vi "trimspace non-reentrant vs reentrant vs inline.vi"() -> ()   [LabVIEW 2020]
panel:
  out "inside 3":i32
  out "[\\t\\n\\r\\s] 2":string
  out "outside 3":i32
  out "[\\t\\n\\r\\s]":string
  out "[\\t\\s]":string
  out "inside 2":i32
  out "outside 2":i32
  out "inside":i32
  out "outside":i32
  out "unit (ms)":dbl[][](graph)
  # "non-reentrant"
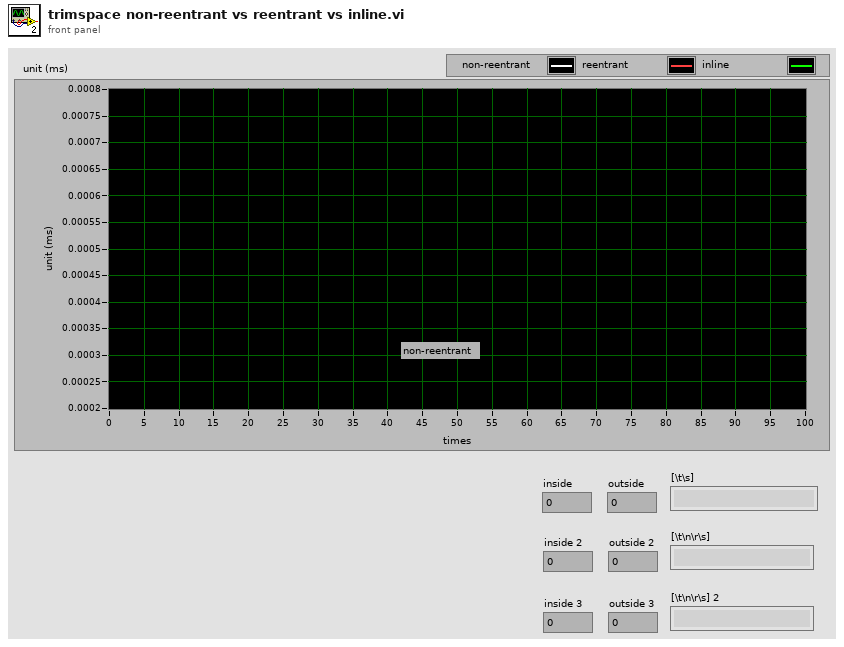
[diagram p1: front panel]
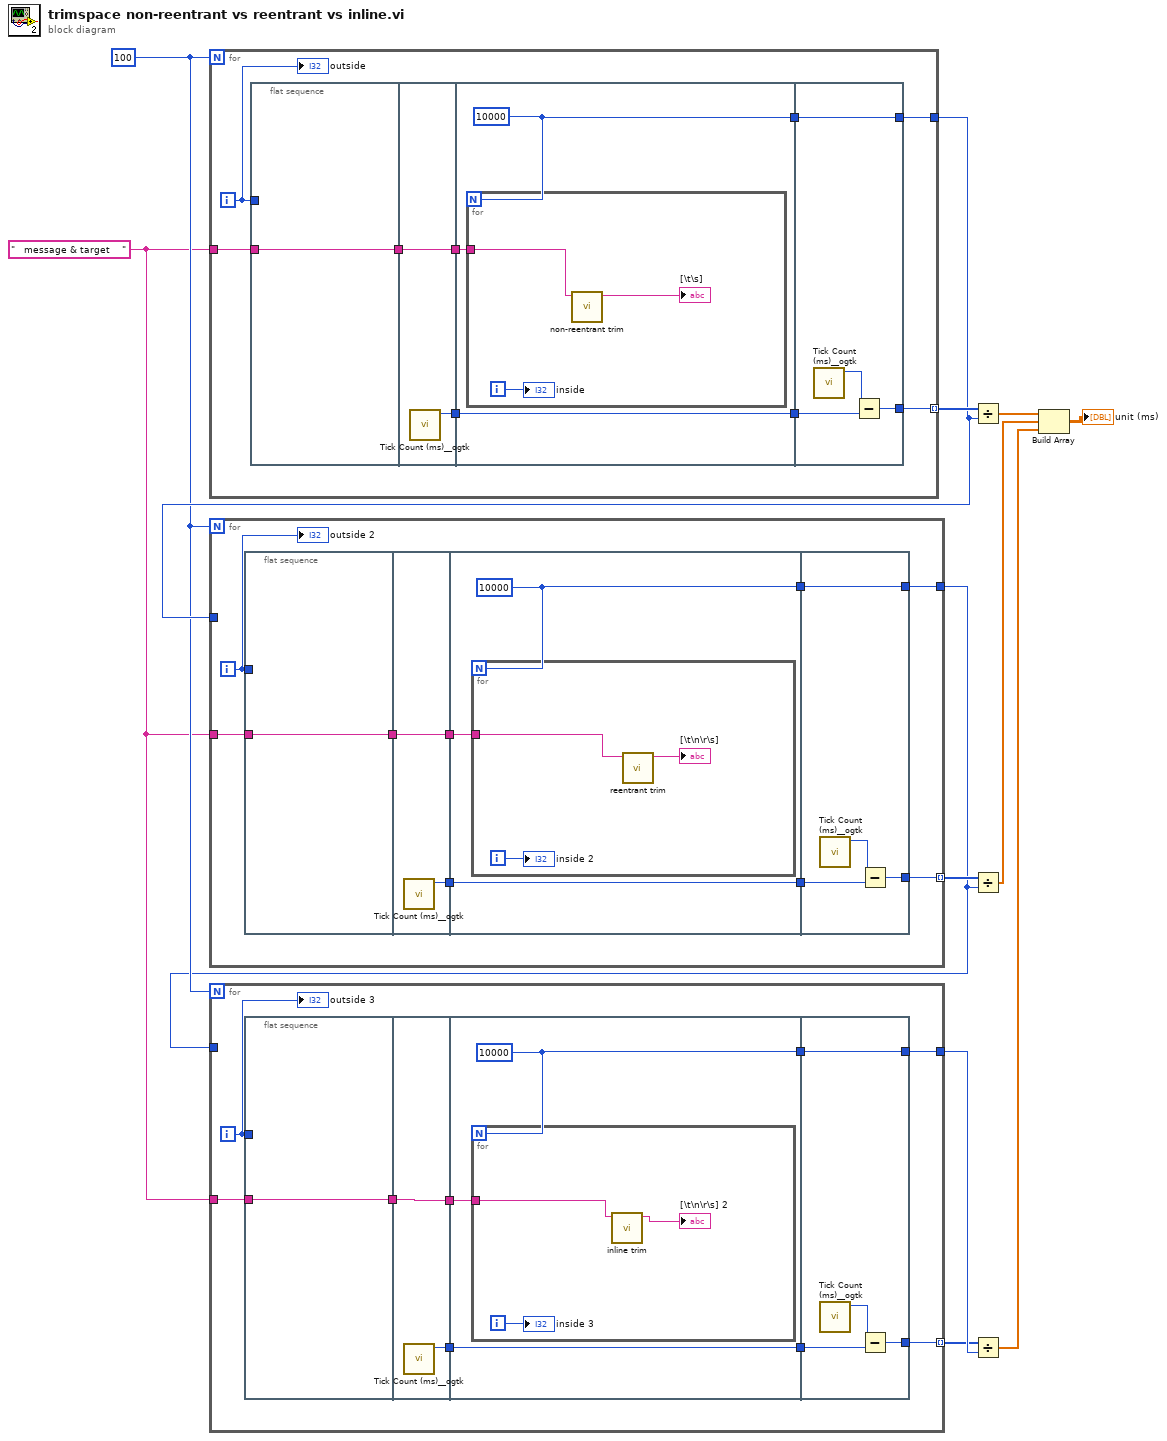
[diagram p0: block diagram]
diagram:
  w2 = "   message & target    " ("string")
  w4 = 100
  n1 = for {
    N: w4 -> [_]
    tunnel: [w19] -> w12 mode=indexing
    tunnel: [w18] -> w9
    tunnel: w2 -> [w13]
    i -> [w16]
    n2 = flat-sequence {
      tunnel: w16 -> [_]
      tunnel: [w22] -> w14
      tunnel: w13 -> [w22]
      tunnel: [w24] -> w21
      tunnel: [w23] -> w15
      tunnel: w14 -> [w23]
      tunnel: w21 -> [w27]
      tunnel: [w27] -> w20
      tunnel: [w26] -> w17
      tunnel: w15 -> [w25]
      tunnel: w20 -> [w33]
      tunnel: [w32] -> w19
      tunnel: [w31] -> w18
      tunnel: w17 -> [w31]
      frame #0 {
      }
      frame #1 {
        n3 = call <userlib>:"Tick Count (ms)__ogtk.vi"() -> ("millisecond timer value"=w24:u32)  [unwired: 10 in, 1 out]
      }
      frame #2 {
        w26 = 10000
        n4 = for {
          N: w26 -> [_]
          tunnel: w25 -> [w29]
          i -> [w30]
          n5 = call "non-reentrant trim.vi"("string in"=w29) -> ("string out"=→"[\\t\\s]":string)  [unwired: 10 in]
          "inside" <- w30
        }
      }
      frame #3 {
        n6 = call <userlib>:"Tick Count (ms)__ogtk.vi"() -> ("millisecond timer value"=w34:u32)  [unwired: 10 in, 1 out]
        n7 = Subtract(x=w34, y=w33) -> (x-y=w32:u32)
      }
    }
    "outside" <- w16
  }
  n8 = for {
    N: w4 -> [_]
    tunnel: [w41] -> w10 mode=indexing
    tunnel: [w40] -> w3
    tunnel: w9 -> [_]
    tunnel: w2 -> [w35]
    i -> [w38]
    n9 = flat-sequence {
      tunnel: w38 -> [_]
      tunnel: [w44] -> w36
      tunnel: w35 -> [w44]
      tunnel: [w46] -> w43
      tunnel: [w45] -> w37
      tunnel: w36 -> [w45]
      tunnel: w43 -> [w49]
      tunnel: [w49] -> w42
      tunnel: [w48] -> w39
      tunnel: w37 -> [w47]
      tunnel: w42 -> [w55]
      tunnel: [w54] -> w41
      tunnel: [w53] -> w40
      tunnel: w39 -> [w53]
      frame #0 {
      }
      frame #1 {
        n10 = call <userlib>:"Tick Count (ms)__ogtk.vi"() -> ("millisecond timer value"=w46:u32)  [unwired: 10 in, 1 out]
      }
      frame #2 {
        w48 = 10000
        n11 = for {
          N: w48 -> [_]
          tunnel: w47 -> [w50]
          i -> [w52]
          n12 = call "reentrant trim.vi"("string in"=w50) -> ("string out"=→"[\\t\\n\\r\\s]":string)  [unwired: 10 in]
          "inside 2" <- w52
        }
      }
      frame #3 {
        n13 = call <userlib>:"Tick Count (ms)__ogtk.vi"() -> ("millisecond timer value"=w56:u32)  [unwired: 10 in, 1 out]
        n14 = Subtract(x=w56, y=w55) -> (x-y=w54:u32)
      }
    }
    "outside 2" <- w38
  }
  n15 = for {
    N: w4 -> [_]
    tunnel: [w63] -> w5 mode=indexing
    tunnel: [w62] -> w6
    tunnel: w2 -> [w57]
    tunnel: w3 -> [_]
    i -> [w60]
    n16 = flat-sequence {
      tunnel: w60 -> [_]
      tunnel: [w66] -> w58
      tunnel: w57 -> [w66]
      tunnel: [w68] -> w65
      tunnel: [w67] -> w59
      tunnel: w58 -> [w67]
      tunnel: w65 -> [w71]
      tunnel: [w71] -> w64
      tunnel: [w70] -> w61
      tunnel: w59 -> [w69]
      tunnel: w64 -> [w77]
      tunnel: [w76] -> w63
      tunnel: [w75] -> w62
      tunnel: w61 -> [w75]
      frame #0 {
      }
      frame #1 {
        n17 = call <userlib>:"Tick Count (ms)__ogtk.vi"() -> ("millisecond timer value"=w68:u32)  [unwired: 10 in, 1 out]
      }
      frame #2 {
        w70 = 10000
        n18 = for {
          N: w70 -> [_]
          tunnel: w69 -> [w72]
          i -> [w74]
          n19 = call "inline trim.vi"("string in"=w72) -> ("string out"=→"[\\t\\n\\r\\s] 2":string)  [unwired: 10 in]
          "inside 3" <- w74
        }
      }
      frame #3 {
        n20 = call <userlib>:"Tick Count (ms)__ogtk.vi"() -> ("millisecond timer value"=w78:u32)  [unwired: 10 in, 1 out]
        n21 = Subtract(x=w78, y=w77) -> (x-y=w76:u32)
      }
    }
    "outside 3" <- w60
  }
  n22 = Divide(x=w12, y=w9) -> (x/y=w7:dbl[])
  n23 = Divide(x=w10, y=w3) -> (x/y=w8:dbl[])
  n24 = Divide(x=w5, y=w6) -> (x/y=w1:dbl[])
  n25 = Build Array(w7, w8, w1) -> (→"unit (ms)":dbl[][])
